vi "ImPro - Gamma Adjustment.vi"(8 "error in (no error)":errorcluster, 10 "24-bit pixmap In":u32[][](array[numeric]), 11 "Brightness (Gamma)":dbl) -> (0 "error out":errorcluster, 2 "24-bit pixmap Out":u32[][](array[numeric]), 3 "R 1D Array":u8[](array[numeric]))   [LabVIEW 2023]
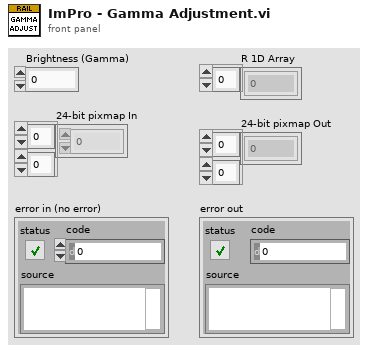
[diagram p1: front panel]
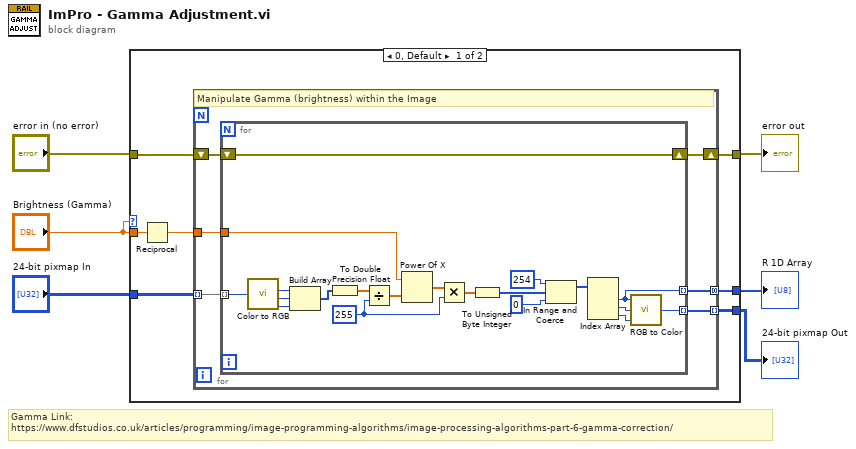
[diagram p0: block diagram]
diagram:
  # "Gamma Link:\nhttps://www.dfstudios.co.uk/articles/programming/image-programming-algorithms/image-processing-algorithms-part-6-gamma-correction/"
  n1 = case shown="0, Default" "Brightness (Gamma)" {
    tunnel: [w13 w40] -> w6
    tunnel: "24-bit pixmap In" -> [w12 w41]
    tunnel: "error in (no error)" -> [w11 w40]
    tunnel: "Brightness (Gamma)" -> [w10 _]
    tunnel: [w9 _] -> w3
    tunnel: [w8 w41] -> w2
    frame 0, Default {
      n2 = Reciprocal(x=w10) -> (1/x=w7:dbl)
      n3 = for {
        tunnel: w12 -> [w19] mode=indexing
        tunnel: w7 -> [w18]
        tunnel: [w17] -> w8 mode=indexing
        tunnel: [w16] -> w9 mode=concatenating
        shift-right: [w15] -> w13
        shift-left: w11 -> [w14]
        # "Manipulate Gamma (brightness) within the Image"
        n4 = for {
          tunnel: w19 -> [w39] mode=indexing
          tunnel: w18 -> [w24]
          tunnel: [w31] -> w17 mode=indexing
          tunnel: [w30] -> w16 mode=indexing
          shift-right: [w20] -> w15
          shift-left: w14 -> [w20]
          w22 = u8 255 ("unsigned 8bit integer")
          n5 = call <vilib>:"Color to RGB.vi"("Color"=w39) -> ("R"=w29:u8, "G"=w38:u8, "B"=w37:u8)  [unwired: 1 out]
          n6 = Build Array(w29, w38, w37) -> (w28:u8[])
          n7 = To Double Precision Float(number=w28) -> (double precision float=w26:dbl[])
          n8 = Divide(x=w26, y=w22) -> (x/y=w25:dbl[])
          n9 = Power Of X(1:w25, 2:w24) -> (0:w23:dbl[])
          n10 = Multiply(x=w23, y=w22) -> (x*y=w21:dbl[])
          n11 = To Unsigned Byte Integer(number=w21) -> (unsigned 8bit integer=w27:u8[])
          n12 = In Range and Coerce(upper limit=u8 254, x=w27, lower limit=u8 0) -> (coerced(x)=w34:u8[])  [unwired: 1 out]
          n13 = Index Array(array=w34) -> (element #1=w30:u8, element #2=w33:u8, element #3=w32:u8)  [unwired: 3 in]
          n14 = call <vilib>:"RGB to Color.vi"("B"=w32, "G"=w33, "R"=w30) -> ("Color"=w31:u32)
        }
      }
    }
    frame 1 {
      # "Do nothing..."
    }
  }
  "error out" <- w6
  "R 1D Array" <- w3
  "24-bit pixmap Out" <- w2
